vi "SetArmTimer.vi"(8 "Error In":errorcluster, 10 "Interval (sec)":dbl, 11 "Keithley 6482 In":refnum<visa-resource-name>) -> (0 "Error Out":errorcluster, 3 "Keithley 6482 Out":refnum<visa-resource-name>)   [LabVIEW 8.6, in "Keithley-6482-Visa.lvlib"]
uses:
  Keithley-6482-Visa.lvlib
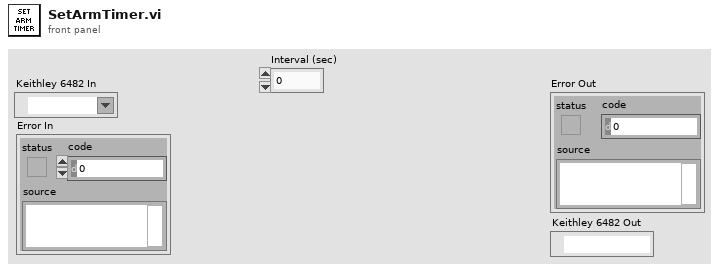
[diagram p1: front panel]
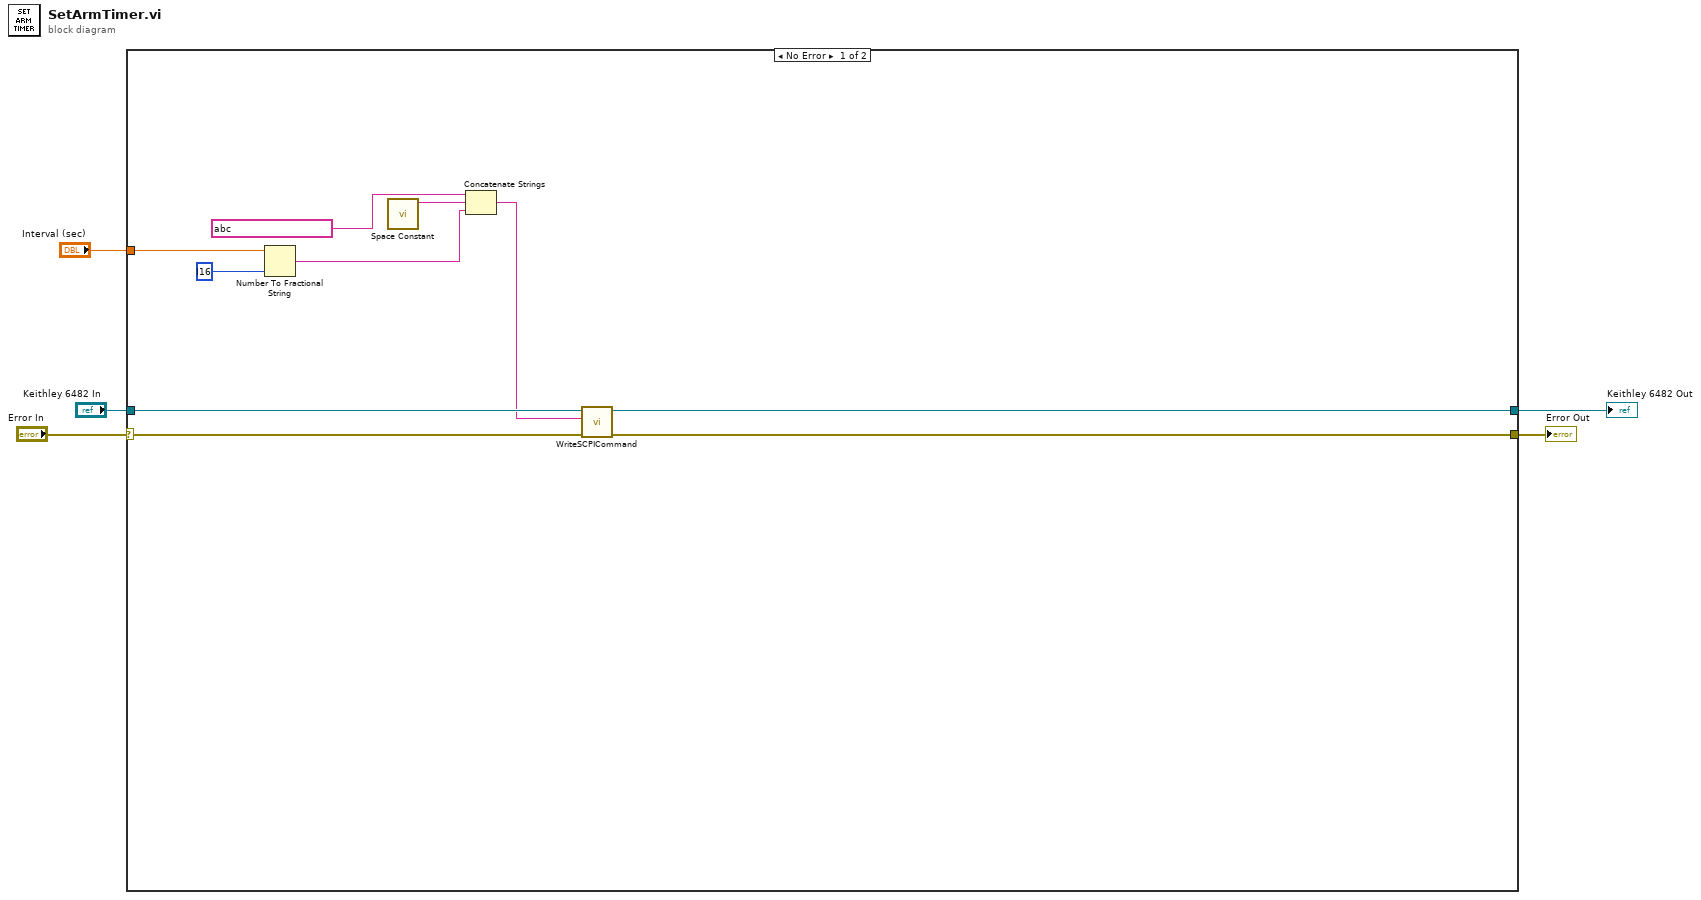
[diagram p0: block diagram]
diagram:
  n1 = case shown="No Error" "Error In" {
    selector: "Error In" -> [w15 w16]
    tunnel: "Keithley 6482 In" -> [w14 w17]
    tunnel: [w9 w16] -> w3
    tunnel: [w10 w17] -> w2
    tunnel: "Interval (sec)" -> [w8 _]
    frame #0 {
      n2 = Number To Fractional String(number=w8, precision (6)=i16 ?) -> (F-format string=w6:string)  [unwired: 2 in]
      n3 = call <vilib>:"Space Constant.vi"() -> ("String"=w12:string)
      n4 = Concatenate Strings(string ? ("string"), w12, w6) -> (w11:string)
      n5 = call "WriteSCPICommand.vi"("Error In"=w15, "SCPI Command"=w11, "Keithley 6482 In"=w14) -> ("Error Out"=w9:errorcluster, "Keithley 6482 Out"=w10:refnum<visa-resource-name>)  [unwired: 7 in]
    }
    frame #1 {
    }
  }
  "Error Out" <- w3
  "Keithley 6482 Out" <- w2
